vi "VI AK Master.vi"(8 "error in (no error)":errorcluster caption="Fehler (Eingang, kein Fehler)") -> (0 "error out":errorcluster)   [LabVIEW 2020, in "FT-IR.lvlib" / "AK-Interface.lvlib"]
uses:
  AK-Interface.lvlib
  Aktionen AK.ctl
  Allgemein/Zykluszeiterfassung Aktionen.ctl
  TCP Timeout Aktionen - FTIR.ctl
  Stoerungen/Stoerungen Messgeraet/Aktionen Kommunikation Stoerung.ctl
  Allgemein/allgemeine Sub-VIs.lvlib
  Stoerungen/Stoerungen.lvlib
panel:
  out "Hz":sgl=80.0 format="%#.1f"
  out "Zustand":T1
  out "initialisieren":errorcluster caption="initiálisieren"
  out "Diagramm":u32(graph)
  out "AK Komm":errorcluster
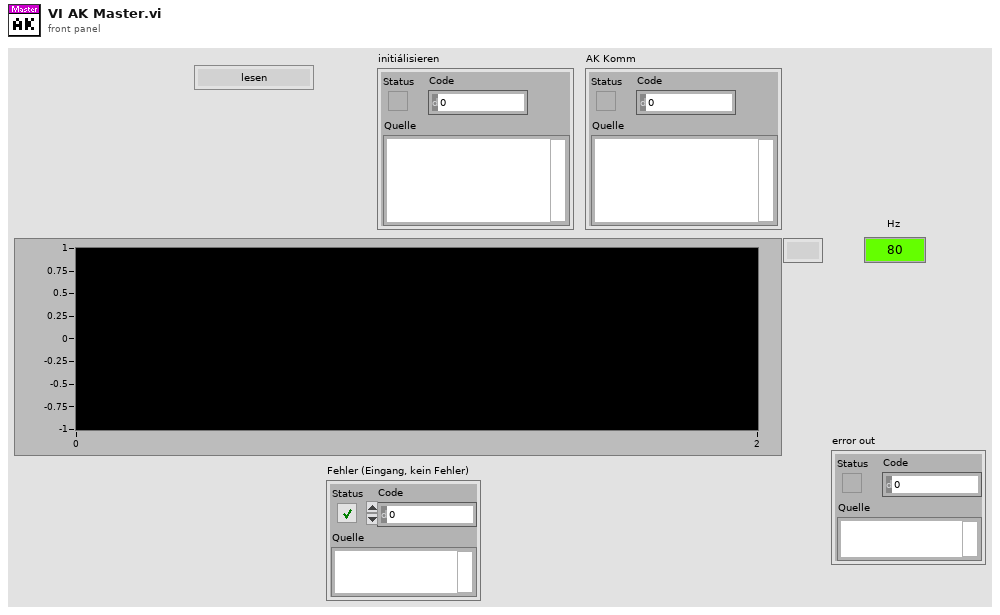
[diagram p1: front panel]
types:
  T1 = typedef "FT-IR.lvlib/AK-Interface.lvlib/Aktionen AK.ctl" = enum16{"lesen", "initialisieren", "beenden", "AK Komm"}
  T2 = typedef "FT-IR.lvlib/AK-Interface.lvlib/TCP Timeout Aktionen - FTIR.ctl" = enum16{"lesen", "setzen"}
  T3 = typedef "allgemeine Sub-VIs.lvlib/Zykluszeiterfassung Aktionen.ctl" = enum16{"lesen", "init", "Messdaten1", "ToolWeb", "AK FT-IR", "AK Extern", "AK Amium"}
  T4 = typedef "Stoerungen.lvlib/Aktionen Kommunikation Stoerung.ctl" = enum16{"lesen", "init", "FT-IR Komm", "FT-IR Betriebsart", "FT-IR Hintergrund", "cRIO Komm", "PNS Komm", "Dichtheitstest", "Life Bit", "FTIR Komm AK", "PMA Komm", "FID Komm", "PMA Cal", "FID Ch4 Cal", "FID THC Cal", "Cal Timeout", "VFS 1 Komm", "VFS 2 Komm", "VFS 3 Komm", "VFS 4 Komm", "TRE 08 Komm", "CG-Test vorzeitig", "CG-Test Span 1", "CG-Test Span 2", "CG-Test Span 3", "CG-Test Messgas", "CG-Test löschen", "Test", "Amium AK", "AK Recept konfig", "AK Name konfig", "AK EKFG konfig"}
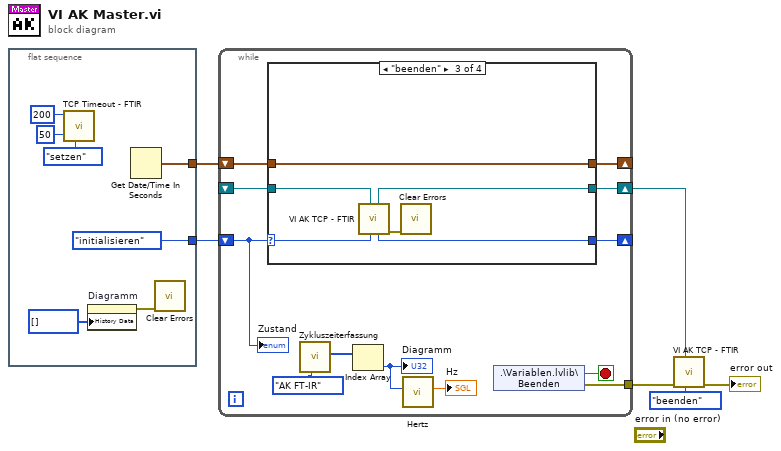
[diagram p0: block diagram]
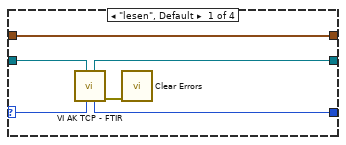
[diagram p2: hidden frame]
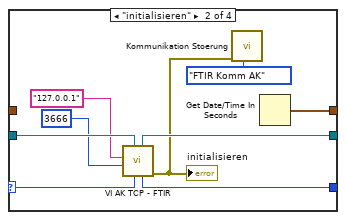
[diagram p3: hidden frame]
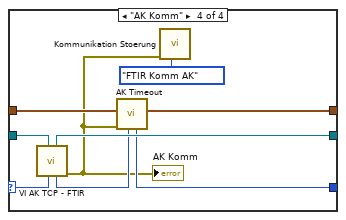
[diagram p4: hidden frame]
diagram:
  n1 = flat-sequence {
    tunnel: [Aktionen_AK."initialisieren" ("Aktionen")] -> w2
    tunnel: [w12] -> w4
    frame #0 {
      n2 = call "TCP Timeout - FTIR.vi"("Aktionen Timeout"=TCP_Timeout_Aktionen_-_FTIR."setzen", "Timeout lesen"=50, "Timeout schreiben"=200) -> ()  [unwired: 7 in, 2 out]
      n3 = property on="Diagramm" class="SVDiagr (strikt)"("History Data"=u32[] [] ("Historiendaten")) -> (error out=w10:errorcluster)  [unwired: 2 in, 1 out]
      n4 = Get Date/Time In Seconds() -> (seconds since 1Jan1904=w12:timestamp)
      n5 = call <vilib>:"Clear Errors.vi"("error in (no error)"=w10) -> ()  [unwired: 5 in, 2 out]
    }
  }
  n6 = while {
    shift-right: [w24] -> _
    shift-left: w2 -> [w25]
    shift-right: [w23] -> _
    shift-left: w4 -> [w22]
    tunnel: [w21] -> w6
    shift-right: [w19] -> w3
    shift-left: _ -> [w18]
    stop <- w20 stop-if-true
    n7 = case shown="\"beenden\"" w25 {
      selector: w25 -> [w30 w40 w46 w52]
      tunnel: [w26 w36 w41 w51] -> w24
      tunnel: [w31 w39 w45 w50] -> w23
      tunnel: w22 -> [w31 _ w45 w55]
      tunnel: [w27 w37 w42 w54] -> w19
      tunnel: w18 -> [w28 w38 w43 w53]
      frame "lesen", Default {
        n8 = call "VI AK TCP - FTIR.vi"("Aktionen"=w30, "connection ID"=w28) -> ("error out"=w29:errorcluster, "Aktionen"=w26:T1, "connection ID"=w27:refnum<k5>)  [unwired: 6 in, 1 out]
        n9 = call <vilib>:"Clear Errors.vi"("error in (no error)"=w29) -> ()  [unwired: 5 in, 2 out]
      }
      frame "initialisieren" {
        n10 = call "VI AK TCP - FTIR.vi"("Aktionen"=w40, "connection ID"=w38, "Port"=u16 3666, "IP-Adresse:"="127.0.0.1" ("IP-Adresse")) -> ("error out"=w32:errorcluster, "Aktionen"=w36:T1, "connection ID"=w37:refnum<k5>)  [unwired: 4 in, 1 out]
        "initialisieren" <- w32
        n11 = call "Kommunikation Stoerung.vi"("Aktionen"=Aktionen_Kommunikation_Stoerung."FTIR Komm AK", "error in"=w32) -> ()  [unwired: 9 in, 1 out]
        n12 = Get Date/Time In Seconds() -> (seconds since 1Jan1904=w39:timestamp)
      }
      frame "beenden" {
        n13 = call "VI AK TCP - FTIR.vi"("Aktionen"=w46, "connection ID"=w43) -> ("error out"=w44:errorcluster, "Aktionen"=w41:T1, "connection ID"=w42:refnum<k5>)  [unwired: 6 in, 1 out]
        n14 = call <vilib>:"Clear Errors.vi"("error in (no error)"=w44) -> ()  [unwired: 5 in, 2 out]
      }
      frame "AK Komm" {
        n15 = call "VI AK TCP - FTIR.vi"("Aktionen"=w52, "connection ID"=w53) -> ("error out"=w48:errorcluster, "Aktionen"=w49:T1, "connection ID"=w54:refnum<k5>)  [unwired: 6 in, 1 out]
        "AK Komm" <- w48
        n16 = call "AK Timeout.vi"("Aktionen"=w49, "Fehler"=w48, "Zeitstempel"=w55) -> ("Zeitstempel"=w50:timestamp, "Aktionen"=w51:T1)  [unwired: 7 in]
        n17 = call "Kommunikation Stoerung.vi"("Aktionen"=Aktionen_Kommunikation_Stoerung."FTIR Komm AK", "error in"=w48) -> ()  [unwired: 9 in, 1 out]
      }
    }
    n18 = call "Zykluszeiterfassung.vi"("Aktionen"=Zykluszeiterfassung_Aktionen."AK FT-IR") -> ("Zykluszeiten"=w16:u32[])  [unwired: 10 in]
    n19 = Index Array(array=w16) -> (element=w15:u32)  [unwired: 1 in]
    "Diagramm" <- w15
    n20 = call "Hertz.vi"("Zeit [ms]"=w15) -> ("Hertz"=→"Hz":sgl)  [unwired: 10 in]
    n21 = shared-variable ".\\Variablen.lvlib\\Beenden"() -> (w20:bool, error out=w21:errorcluster)  [unwired: 1 in]
    "Zustand" <- w25
  }
  n22 = call "VI AK TCP - FTIR.vi"("Aktionen"=Aktionen_AK."beenden", "connection ID"=w3, "error in"=w6) -> ("error out"=→"error out":errorcluster)  [unwired: 5 in, 3 out]
